vi "Core Recieve Message.vi"(7 "Message Priority":T1=enum."Normal", 8 "error in (no error)":errorcluster, 9 "Message in":refnum<class "Message.lvclass">, 10 "Actor in":refnum<class "Actor.lvclass">, 11 "Multi Instrument Sequencer":refnum<class "Multi Instrument Sequencer.lvclass">) -> (0 "error out":errorcluster, 2 "Actor out":refnum<class "Actor.lvclass">, 3 "Multi Instrument Sequencer":refnum<class "Multi Instrument Sequencer.lvclass">)   [LabVIEW 2020, in "Instrument Handler.lvlib" / "Multi Instrument Sequencer.lvclass"]
doc: "This implementation forwards Instrument Msgs to the other instrument processes where they are executed."
uses:
  Multi Instrument Sequencer.lvclass
  PPL/HDH.Actor Framework.Core.Actor.lvlibp/1abvi3w/vi.lib/ActorFramework/Message/Message.lvclass
  PPL/HDH.Actor Framework.Core.Actor.lvlibp/1abvi3w/vi.lib/ActorFramework/Actor/Actor.lvclass
  PPL/HDH.Actor Framework.Core.Actor.lvlibp/1abvi3w/vi.lib/ActorFramework/Message Enqueuer/Message Priority.ctl
  Messages/Multi Instrument Wrapper Msg/Multi Instrument Wrapper Msg.lvclass
  Multi Instrument Handler/Multi Instrument Handler.lvclass
  C:/Current projects/WS/PPL/HDH.Actor Framework.Core.Actor.lvlibp/1abvi3w/vi.lib/ActorFramework/Actor/Actor.lvclass
  Messages/Multi Instrument Wrapper Msg/Multi Instrument Wrapper Msg.lvclass/Multi Instrument Wrapper Msg.ctl
  Multi Instrument Handler/Multi Instrument Handler.lvclass/Multi Instrument Handler.ctl
  Messages/Release Aquirer Msg/Release Aquirer Msg.lvclass/Release Aquirer Msg.ctl
  Instrument Handler Messages/Decrement Multi Instrument Handler Msg/Decrement Multi Instrument Handler Msg.lvclass/Decrement Multi Instrument Handler Msg.ctl
  Messages/Multi Instrument Msg/Multi Instrument Msg.lvclass
  C:/Current projects/WS/Framework/Framework/Actors/Instrument Handler/Messages/Instrument Msg/Instrument Msg.lvclass
  PPL/HDH.Actor Framework.Core.Actor.lvlibp/1abvi3w/vi.lib/ActorFramework/Actor/Read Caller Enqueuer.vi
  PPL/HDH.Actor Framework.Core.Actor.lvlibp/1abvi3w/vi.lib/ActorFramework/Message Enqueuer/Enqueue.vi
  PPL/HDH.Actor Framework.Core.Actor.lvlibp/1abvi3w/vi.lib/ActorFramework/Message Enqueuer/Message Enqueuer.lvclass
  Messages/Release Aquirer Msg/Release Aquirer Msg.lvclass
  Instrument Handler Messages/Decrement Multi Instrument Handler Msg/Decrement Multi Instrument Handler Msg.lvclass
  PPL/HDH.Actor Framework.Core.Sequencer.lvlibp/Sequencer Core/Sequencer Core.lvclass
  PPL/HDH.Actor Framework.Core.Publisher.lvlibp/Messages/Response Msg/Response Msg.lvclass
  Messages/Instrument Msg/Instrument Msg.lvclass
  Instrument Handler.lvlib
  C:/Current projects/WS/PPL/HDH.Actor Framework.Core.Publisher.lvlibp/Messages/Response Msg/Response Msg.lvclass
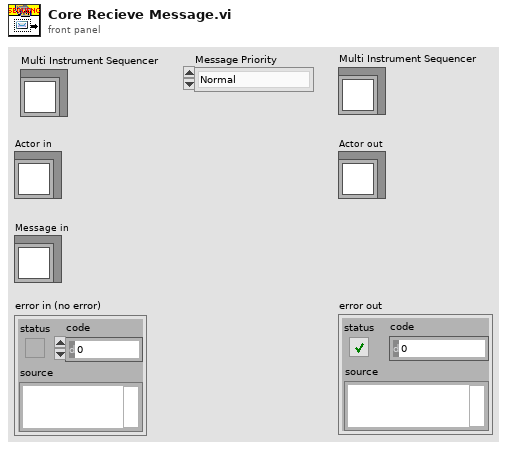
[diagram p1: front panel]
types:
  T1 = typedef "HDH.Actor Framework.Core.Actor.lvlibp/Message Enqueuer.lvclass/Message Priority.ctl" = enum16{"Low", "Normal", "High"}
  T2 = typedef "Instrument Handler.lvlib/Ctl_AquirerRefnum.ctl" = refnum<vi>
  T3 = typedef "Semaphore RefNum" = refnum<k1>
  T4 = typedef "Instrument Handler.lvlib/Ctl_AquirerCompletionStatus.ctl" = cluster{"Success?":bool, "Aquirer Index":i32}
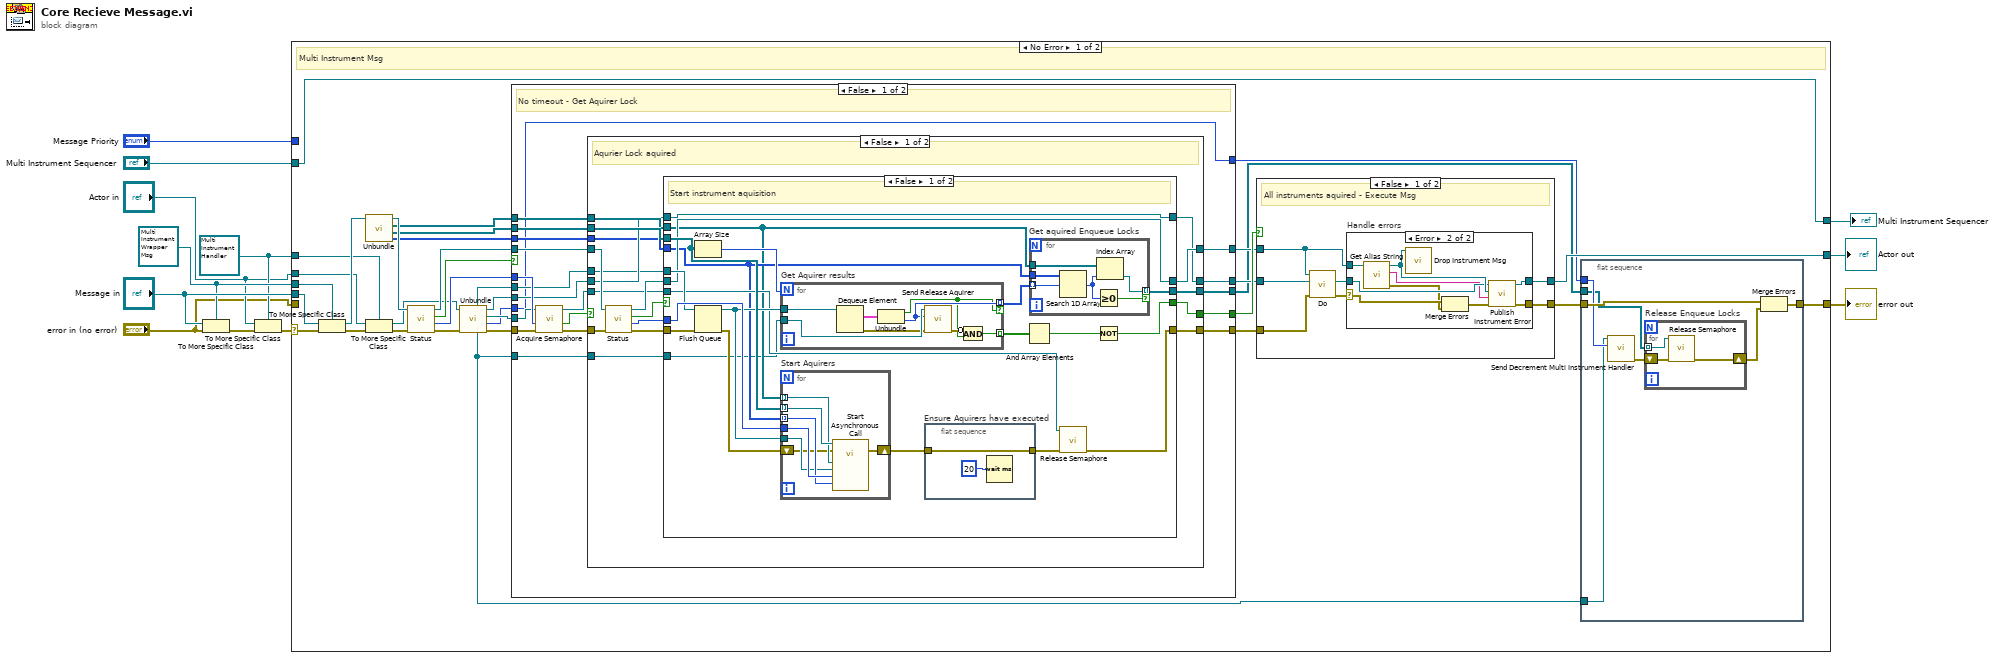
[diagram p0: block diagram]
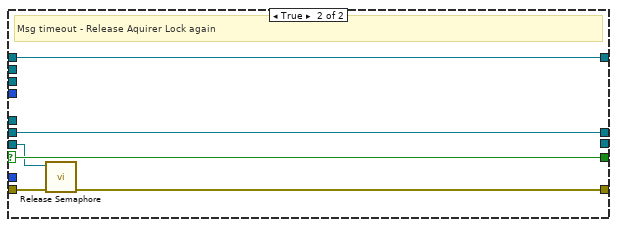
[diagram p2: hidden frame]
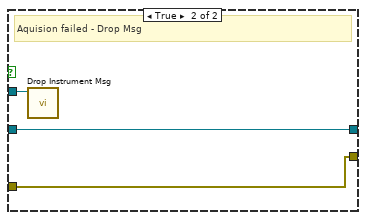
[diagram p6: hidden frame]
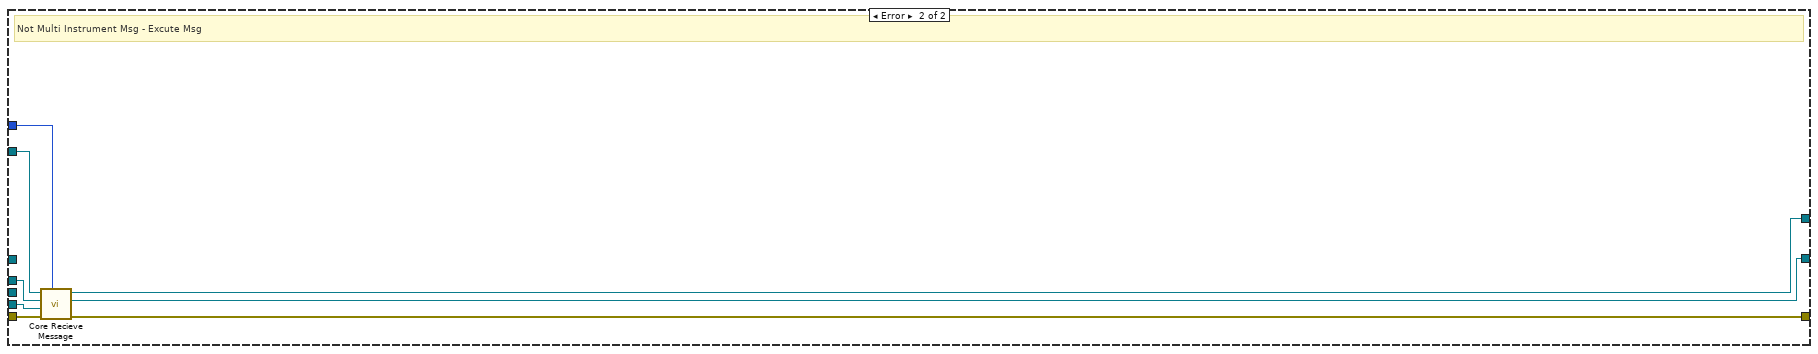
[diagram p7: hidden frame]
diagram:
  w6 = refnum<class "Multi Instrument Handler.lvclass"> refnum ("Instrument Handler in")
  w9 = refnum<class "Multi Instrument Wrapper Msg.lvclass"> refnum ("Instrument Handler.lvlib:Multi Instrument Wrapper Msg.lvclass")
  n1 = To More Specific Class(target class=w9, reference="Message in", error in="error in (no error)") -> (error out=w8:errorcluster)  [unwired: 1 out]
  n2 = To More Specific Class(target class=w6, reference="Actor in", error in=w8) -> (error out=w7:errorcluster)  [unwired: 1 out]
  n3 = case shown="No Error" w7 {
    selector: w7 -> [w44 _]
    tunnel: [w27 w177] -> w12
    tunnel: [w29 w179] -> w11
    tunnel: "Message Priority" -> [_ w173]
    tunnel: "Message in" -> [w45 w174]
    tunnel: w9 -> [w43 _]
    tunnel: w6 -> [w16 _]
    tunnel: "Actor in" -> [w14 w180]
    tunnel: [w13 w176] -> w3
    tunnel: "Multi Instrument Sequencer" -> [w13 w175]
    tunnel: "error in (no error)" -> [_ w178]
    frame No Error {
      # "Multi Instrument Msg"
      n4 = To More Specific Class(target class=w43, reference=w45, error in=w44) -> (specific class reference=w42:refnum<class "Multi Instrument Wrapper Msg.lvclass">, error out=w18:errorcluster)
      n5 = call "Unbundle.vi"("Multi Instrument Wrapper Msg in"=w42) -> ("Aquirer Indices"=w31:i32[], "Aquirer"=w33:T2[], "Enqueue Locks"=w32:T3[], "Msg"=w41:refnum<class "Multi Instrument Msg.lvclass">)  [unwired: 7 in]
      n6 = To More Specific Class(target class=w16, reference=w14, error in=w18) -> (specific class reference=w15:refnum<class "Multi Instrument Handler.lvclass">, error out=w17:errorcluster)
      n7 = call "Status.vi"("error in (no error)"=w17, "Response Msg in"=w41) -> ("error out"=w21:errorcluster, "Time to Timeout (ms)"=w40:i32, "Dropped?"=w39:bool, "Response Msg out"=w36:refnum<class "Multi Instrument Msg.lvclass">)  [unwired: 6 in]
      n8 = call "Unbundle.vi"("error in (no error)"=w21, "Multi Instrument Handler in"=w15) -> ("error out"=w20:errorcluster, "Hander Index"=w23:i32, "Aquirer Lock"=w24:T3, "Multi Instrument Handler out"=w22:refnum<class "Multi Instrument Handler.lvclass">, "Caller Enqueuer"=w19:refnum<class "Message Enqueuer.lvclass">, "Aquisition queue"=w25:refnum<queue>)  [unwired: 4 in]
      n9 = case shown="False" w39 {
        selector: w39 -> [_ w151]
        tunnel: w40 -> [w74 _]
        tunnel: w20 -> [w73 w149]
        tunnel: [w68 w151] -> w38
        tunnel: [w70 w150] -> w37
        tunnel: w36 -> [w69 w150]
        tunnel: [w67 w149] -> w35
        tunnel: [w71 w148] -> w30
        tunnel: w22 -> [w61 w148]
        tunnel: w33 -> [w64 _]
        tunnel: w32 -> [w63 _]
        tunnel: w31 -> [w62 _]
        tunnel: [w57 w147] -> w28
        tunnel: [w60 _] -> w26
        tunnel: w25 -> [w59 _]
        tunnel: w24 -> [w58 _]
        tunnel: w23 -> [w57 w147]
        tunnel: w19 -> [w56 _]
        frame False {
          # "No timeout - Get Aquirer Lock"
          n10 = call <vilib>:"Acquire Semaphore.vi"("error in (no error)"=w73, "ms timeout (-1)"=w74, "semaphore"=w58) -> ("error out"=w66:errorcluster, "timed out"=w72:bool, "semaphore out"=w65:T3)  [unwired: 2 in]
          n11 = case shown="False" w72 {
            selector: w72 -> [_ w144]
            tunnel: [w84 w146] -> w71
            tunnel: w61 -> [w83 w146]
            tunnel: [w86 w145] -> w70
            tunnel: w69 -> [w90 w145]
            tunnel: [w87 w144] -> w68
            tunnel: [w78 w143] -> w67
            tunnel: w66 -> [w89 w143]
            tunnel: w65 -> [w77 _]
            tunnel: w64 -> [w92 _]
            tunnel: w63 -> [w91 _]
            tunnel: w62 -> [w80 _]
            tunnel: w59 -> [w79 _]
            tunnel: [w76 _] -> w60
            tunnel: w56 -> [w75 _]
            frame False {
              # "Aqurier Lock aquired"
              n12 = call "Status.vi"("error in (no error)"=w89, "Response Msg in"=w90) -> ("error out"=w82:errorcluster, "Time to Timeout (ms)"=w81:i32, "Dropped?"=w88:bool, "Response Msg out"=w85:refnum<class "Multi Instrument Msg.lvclass">)  [unwired: 6 in]
              n13 = case shown="False" w88 {
                selector: w88 -> [_ w142]
                tunnel: w92 -> [w112 _]
                tunnel: w91 -> [w96 _]
                tunnel: [w105 w142] -> w87
                tunnel: [w104 w141] -> w86
                tunnel: w85 -> [w104 w141]
                tunnel: [w93 w140] -> w84
                tunnel: w83 -> [w93 w140]
                tunnel: [w103 w137] -> w78
                tunnel: w82 -> [w110 w138]
                tunnel: w81 -> [w113 _]
                tunnel: w80 -> [w97 _]
                tunnel: w79 -> [w108 _]
                tunnel: w77 -> [w102 w139]
                tunnel: [w95 _] -> w76
                tunnel: w75 -> [w94 _]
                frame False {
                  # "Start instrument aquisition"
                  n14 = Array Size(array=w112) -> (size(s)=w111:i32)
                  n15 = Flush Queue(queue=w108, error in (no error)=w110) -> (queue out=w107:refnum<queue>, error out=w109:errorcluster)  [unwired: 1 out]
                  n16 = for "Get Aquirer results" {
                    N: w111 -> [_]
                    tunnel: w94 -> [w128]
                    tunnel: [w126] -> w106 mode=indexing
                    tunnel: w107 -> [w125]
                    tunnel: [w123] -> w98 mode=indexing if=w122
                    n17 = Dequeue Element(queue=w125) -> (element=w129:T4, error out=w124:errorcluster)  [unwired: 2 in, 2 out]
                    n18 = Unbundle(w129) -> ("Success?"=w122:bool, "Aquirer Index"=w123:i32)
                    n19 = call "Send Release Aquirer.vi"("error in (no error)"=w124, "Aquirer Index"=w123, "Message Enqueuer"=w128) -> ("error out"=w127:errorcluster)  [unwired: 8 in]
                    n20 = Compound Arithmetic op=AND(invert w127, w122) -> (w126:bool)
                  }
                  n21 = for "Start Aquirers" {
                    tunnel: w112 -> [w136] mode=indexing
                    tunnel: w96 -> [w135] mode=indexing
                    tunnel: w113 -> [w134]
                    tunnel: w97 -> [w133] mode=indexing
                    tunnel: w107 -> [w132]
                    shift-right: [w130] -> w100
                    shift-left: w109 -> [w131]
                    n22 = call-by-ref "Start Asynchronous Call"(reference=w136, error in=w131, "Aquirer Index"=w133, "Timeout(-1ms)"=w134, "Aquirer Queue"=w132, "Enqueue Lock"=w135) -> (error out=w130:errorcluster)  [unwired: 8 in, 1 out]
                  }
                  n23 = flat-sequence "Ensure Aquirers have executed" {
                    tunnel: [w121] -> w101
                    tunnel: w100 -> [w121]
                    frame #0 {
                      n24 = Wait (ms)(milliseconds to wait=u32 20) -> ()  [unwired: 1 out]
                    }
                  }
                  n25 = And Array Elements(Boolean array=w106) -> (logical AND=w99:bool)
                  n26 = for "Get aquired Enqueue Locks" {
                    tunnel: w98 -> [w118] mode=indexing
                    tunnel: w97 -> [w119]
                    tunnel: w96 -> [w117]
                    tunnel: [w115] -> w95 mode=indexing if=w114
                    n27 = Search 1D Array(1D array=w119, element=w118) -> (index of element=w116:i32)  [unwired: 1 in]
                    n28 = Greater Or Equal To 0?(x=w116) -> (x >= 0?=w114:bool)
                    n29 = Index Array(array=w117, index=w116) -> (element=w115:T3)
                  }
                  n30 = call <vilib>:"Release Semaphore.vi"("error in (no error)"=w101, "semaphore"=w102) -> ("error out"=w103:errorcluster)  [unwired: 4 in, 1 out]
                  n31 = Not(x=w99) -> (.not. x?=w105:bool)
                }
                frame True {
                  # "Msg timeout - Release Aquirer Lock again"
                  n32 = call <vilib>:"Release Semaphore.vi"("error in (no error)"=w138, "semaphore"=w139) -> ("error out"=w137:errorcluster)  [unwired: 4 in, 1 out]
                }
              }
            }
            frame True {
              # "Timeout when getting Aquirer Lock - Drop Msg"
            }
          }
        }
        frame True {
          # "Timeout from start - Drop Msg"
        }
      }
      n33 = case "Drop Msg" shown="False" w38 {
        tunnel: w37 -> [w154 w172]
        tunnel: w35 -> [w157 w170]
        tunnel: [w155 w170] -> w34
        tunnel: [w153 w171] -> w29
        tunnel: w30 -> [w158 w171]
        frame False {
          # "All instruments aquired - Execute Msg"
          n34 = call-dynamic "Do.vi"("error in (no error)"=w157, "Actor in"=w158, "Instrument Msg"=w154) -> ("error out"=w156:errorcluster, "Actor out"=w152:refnum<class "Actor.lvclass">)  [unwired: 7 in]
          n35 = case "Handle errors" shown="Error" w156 {
            selector: w156 -> [w160 w168]
            tunnel: [w160 w161] -> w155
            tunnel: w154 -> [_ w169]
            tunnel: [w159 w165] -> w153
            tunnel: w152 -> [w159 w166]
            frame No Error {
            }
            frame Error {
              n36 = call "Get Alias String.vi"("Multi Instrument Msg in"=w169) -> ("error out"=w162:errorcluster, "Instrument List"=w164:string, "Multi Instrument Msg out"=w167:refnum<class "Multi Instrument Msg.lvclass">)  [unwired: 8 in]
              n37 = call "Drop Instrument Msg.vi"("Instrument Msg in"=w167) -> ()  [unwired: 11 in]
              n38 = Merge Errors(w168, w162) -> (w163:errorcluster)
              n39 = call "Publish Instrument Error.vi"("error in (no error)"=w163, "Instrument String"=w164, "Instrument Msg"=w167, "Actor in"=w166) -> ("error out"=w161:errorcluster, "Actor out"=w165:refnum<class "Actor.lvclass">)  [unwired: 6 in]
            }
          }
        }
        frame True {
          # "Aquision failed - Drop Msg"
          n40 = call "Drop Instrument Msg.vi"("Instrument Msg in"=w172) -> ()  [unwired: 11 in]
        }
      }
      n41 = flat-sequence {
        tunnel: w34 -> [w52]
        tunnel: w28 -> [w51]
        tunnel: [w50] -> w27
        tunnel: w26 -> [w49]
        tunnel: w19 -> [w46]
        frame #0 {
          n42 = call "Send Decrement Multi Instrument Handler.vi"("Hander Index"=w51, "Message Enqueuer"=w46) -> ("error out"=w48:errorcluster)  [unwired: 9 in]
          n43 = for "Release Enqueue Locks" {
            tunnel: w49 -> [w55] mode=indexing
            shift-right: [w53] -> w47
            shift-left: w48 -> [w54]
            n44 = call <vilib>:"Release Semaphore.vi"("error in (no error)"=w54, "semaphore"=w55) -> ("error out"=w53:errorcluster)  [unwired: 4 in, 1 out]
          }
          n45 = Merge Errors(w52, w47) -> (w50:errorcluster)
        }
      }
    }
    frame Error {
      # "Not Multi Instrument Msg - Excute Msg"
      n46 = call-parent "Core Recieve Message.vi"("Message Priority"=w173, "error in (no error)"=w178, "Message"=w174, "Actor in"=w180, "Sequencer Core in"=w175) -> ("error out"=w177:errorcluster, "Actor out"=w179:refnum<class "Actor.lvclass">, "Sequencer Core out"=w176:refnum<class "Multi Instrument Sequencer.lvclass">)  [unwired: 4 in]
    }
  }
  "error out" <- w12
  "Actor out" <- w11
  "Multi Instrument Sequencer" <- w3
